vi "MLP_PID_Trajectory tracking_0128.vi"() -> ()   [LabVIEW 2018]
doc: "Demonstrates the use of the Network Streams functions to send LED status to the myRIO target."
uses:
  <vilib>/ErrorRing/Error Ring.xnode
  <vilib>/vision/NI_Vision_Development_Module.lvlib
panel:
  in  "Operation":T1(ring)=enum."Erode"
  out "real_relative_point_y":dbl
  out "real_relative_point_x":dbl
  out "real_relative_start_point_y":dbl
  out "real_relative_start_point_x":dbl
  out "Bounding Box.Y Top 2":i32
  out "Bounding Box.X Left 2":i32
  out "Ki part":dbl
  out "Kd part":dbl
  out "Kp part":dbl
  out "Ki part":dbl
  out "Kd part":dbl
  out "Kp part":dbl
  in  "Ki":dbl=0.02
  in  "Kd":dbl=1e-05
  in  "Kp":dbl=0.003
  in  "Ki":dbl=0.02
  in  "Kd":dbl=1e-05
  in  "Kp":dbl=0.008
  out "添加的数组":dbl[](array[numeric])
  out "desired_relative_point_y":dbl
  out "desired_relative_point_x":dbl
  out "predicted_output_pr":dbl
  out "predicted_output_dr":dbl
  out "error_relative_point_y":dbl
  out "error_relative_point_x":dbl
  out "real_relative_end_point_y":dbl
  out "real_relative_end_point_x":dbl
  out "magnet_input_pr":dbl
  out "magnet_input_dr":dbl
  in  "打开仅尖端轨迹":bool
  out "仅尖端轨迹":T2(plugin-control)
  out "Bounding Box.Y Top":i32
  out "Bounding Box.X Left":i32
  out "curve_min_y":dbl
  out "curve_min_x":dbl
  out "curve_max_y":dbl
  out "curve_max_x":dbl
  out "relative_end_point_y":dbl
  out "relative_end_point_x":dbl
  out "delta_y":dbl
  out "delta_x":dbl
  out "pr":dbl
  out "tan(v)":dbl
  out "delta_velocity":dbl format="%#_10g"
  out "delta_time":dbl
  out "now time":timestamp[](array[timestamp])
  out "prev time":timestamp[](array[timestamp])
  out "delta_distance":dbl
  out "prev_end_point_y":dbl
  out "prev_end_point_x":dbl
  out "now_end_point_y":dbl
  out "now_end_point_x":dbl
  out "prev_end_point_y":dbl[](array[numeric])
  out "prev_end_point_x":dbl[](array[numeric])
  out "dr":dbl
  in  "Ar":sgl=11.0
  out "all parameters":dbl[][](array[numeric])
  out "direction angle":sgl[](array[numeric])
  out "dr":sgl
  out "strength":dbl[](array[numeric])
  out "场强":dbl
  out "end_point_y":T3
  out "end_point_x":dbl[](array[numeric])
  out "start_point_y":dbl[](array[numeric])
  out "start_point_x":dbl[](array[numeric])
  out "T":i32[](array[numeric])
  out "c":dbl[](array[numeric])
  out "b":dbl[](array[numeric])
  out "a\na":dbl[](array[numeric])
  out "c":dbl
  out "b":dbl
  out "a":dbl
  out "Angles (deg)":sgl[](array[numeric]) format="%.2f"
  in  "wr":sgl
  in  "打开轨迹":bool
  out "中心轨迹和尖端轨迹":T2(plugin-control)
  out "end_y":dbl
  out "end_x":dbl
  out "start_y":dbl
  out "start_x":dbl
  out "Image Pixels (U8)":u8[][](array[numeric])
  in  "Poly":dbl
  out "中心轨迹":T2(plugin-control)
  in  "保存按钮":bool
  out "Object Center":cluster{"X":sgl, "Y":sgl}
  out "黑白图":T2(plugin-control)
  in  "Number of Erosion":i32=5
  in  "Settings":T4={"Objects"=1, "Threshold"=128, "Reject Border"=FALSE, "Fill Holes"=FALSE, "Min Object Size"=TRUE, "Min Size"=5500, "Max Object Size"=FALSE, "Max Size"=100, "Show Search Area"=TRUE, "Show Center"=TRUE, "Show Bounding Box"=TRUE} {"Objects" items=["Bright Objects", "Dark Objects"]; "Threshold" min=1 max=999999999 step=1; "Max Size" min=1 max=999999999 step=1; "Min Size" min=1 max=999999999 step=1}
  out "Objects":T5(array[cluster]) {"Aspect Ratio" format="%.2f"; "Orientation" format="%.2f"; "Area" format="%.2f"; "Object Center"."Y" format="%.2f"; "Object Center"."X" format="%.2f"}
  in  "Search Rect (entire image)":T6={"Left"=160, "Top"=740, "Right"=1900, "Bottom"=1620, "Rotation"=0.0} {"Rotation" format="%.2f"; "Left" scale=0.0..1024.0; "Right" scale=0.0..1024.0}
  in  "Range":cluster{"Lower value":sgl, "Upper value":sgl}={"Lower value"=170.0, "Upper value"=255.0} {"Upper value" format="%.2f"; "Lower value" format="%.2f"}
  out "原图":T2(plugin-control)
  in  "停止":bool
  out "T":i32
  out "T":i32
  in  "磁场变换":bool=TRUE
  in  "Pause":bool
  out "Array":dbl[](array[numeric])
  in  "Parameter Settings":T7(tab)=enum."Rotating Field" caption="Field Types"
  in  "Ag":dbl
  in  "dg":dbl
  in  "pg":dbl
  in  "fg":dbl
  in  "AoOF":dbl
  in  "fo":sgl
  in  "do":sgl
  in  "oo":sgl
  in  "po":sgl
  in  "cc":sgl
  in  "pc":sgl
  in  "wc":sgl
  in  "dc":sgl
  in  "Ac":dbl
  in  "Dis phase step":dbl
  in  "Dis phase frequency (Hz)":dbl
  in  "Dis tumbling frequency (Hz)":dbl
  in  "Dis strength(mT)":dbl
  in  "Swa strength (mT)":dbl
  in  "Swa frequency (Hz)":dbl
  in  "Swa pitch angle (deg)":dbl
  in  "Swa direction angle (deg)":dbl
  in  "Swa ratio":dbl=1.0
  in  "Pitch Angle (rotating around Constant, deg)":dbl
  in  "Ratio (A/C)":sgl
  in  "Direction Angle (deg)":sgl
  in  "Pitch Angle (rotating around Origin, deg)":sgl
  in  "Frequency (Hz)":sgl
  in  "Strength (mT)":dbl
  in  "Ar 2":dbl caption="Ar"
  in  "ratio":sgl
  in  "pr  2":sgl
  in  "dr  2":sgl
  in  "wr  2":sgl
  in  "p_x":sgl
  out "Numeric 5":i32
  in  "Stop":bool
  out "error out":errorcluster
  in  "Target IP Address":string="172.22.11.2"
  # "Overview: Magnetic field calculation, and send parameters to myRIO\nInstructions:\n1. Verify the value of Target IP Address. Set Visa resource name.\n2. Ensure RT Main.vi is already running. \n3. Run this VI. Set parameters of magnetic field."
  # "Strength (mT)"
  # "Frequency (Hz)"
  # "Pitch Angle (deg)"
  # "Direction Angle (deg)"
  # "Strength (mT)"
  # "Pitch Angle (deg)"
  # "Direction Angle (deg)"
  # "Frequency (Hz)"
  # "Strength (mT)"
  # "Oscilation Frequency (Hz)"
  # "Oscilation Angle (deg)"
  # "Pitch Angle (deg)"
  # "Direction Angle (deg)"
  # "Strength (mT)"
  # "Frequency (Hz)"
  # "Pitch Angle (deg)"
  # "Direction Angle (deg)"
  # "Conical Angle (deg)"
  # "Strength (mT)"
  # "Tumbling Frequency (Hz)"
  # "Phase Frequency (Hz)"
  # "Phase Step"
  # "Strength (mT)"
  # "Frequency (Hz)"
  # "Pitch Angle (deg)"
  # "Direction Angle (deg)"
  # "Ratio"
  # "Strength (mT)"
  # "Frequency (Hz)"
  # "Ratio (A/C)"
  # "Direction Angle (deg)"
  # "Pitch Angle (rotating around Origin, deg)"
  # "Pitch Angle (rotating around Constant, deg)"
  # "Strength (mT)"
  # "Frequency (Hz)"
  # "Pitch Angle Y (deg)"
  # "Pitch Angle X (deg)"
  # "Direction Angle (deg)"
  # "ratio (l/s)"
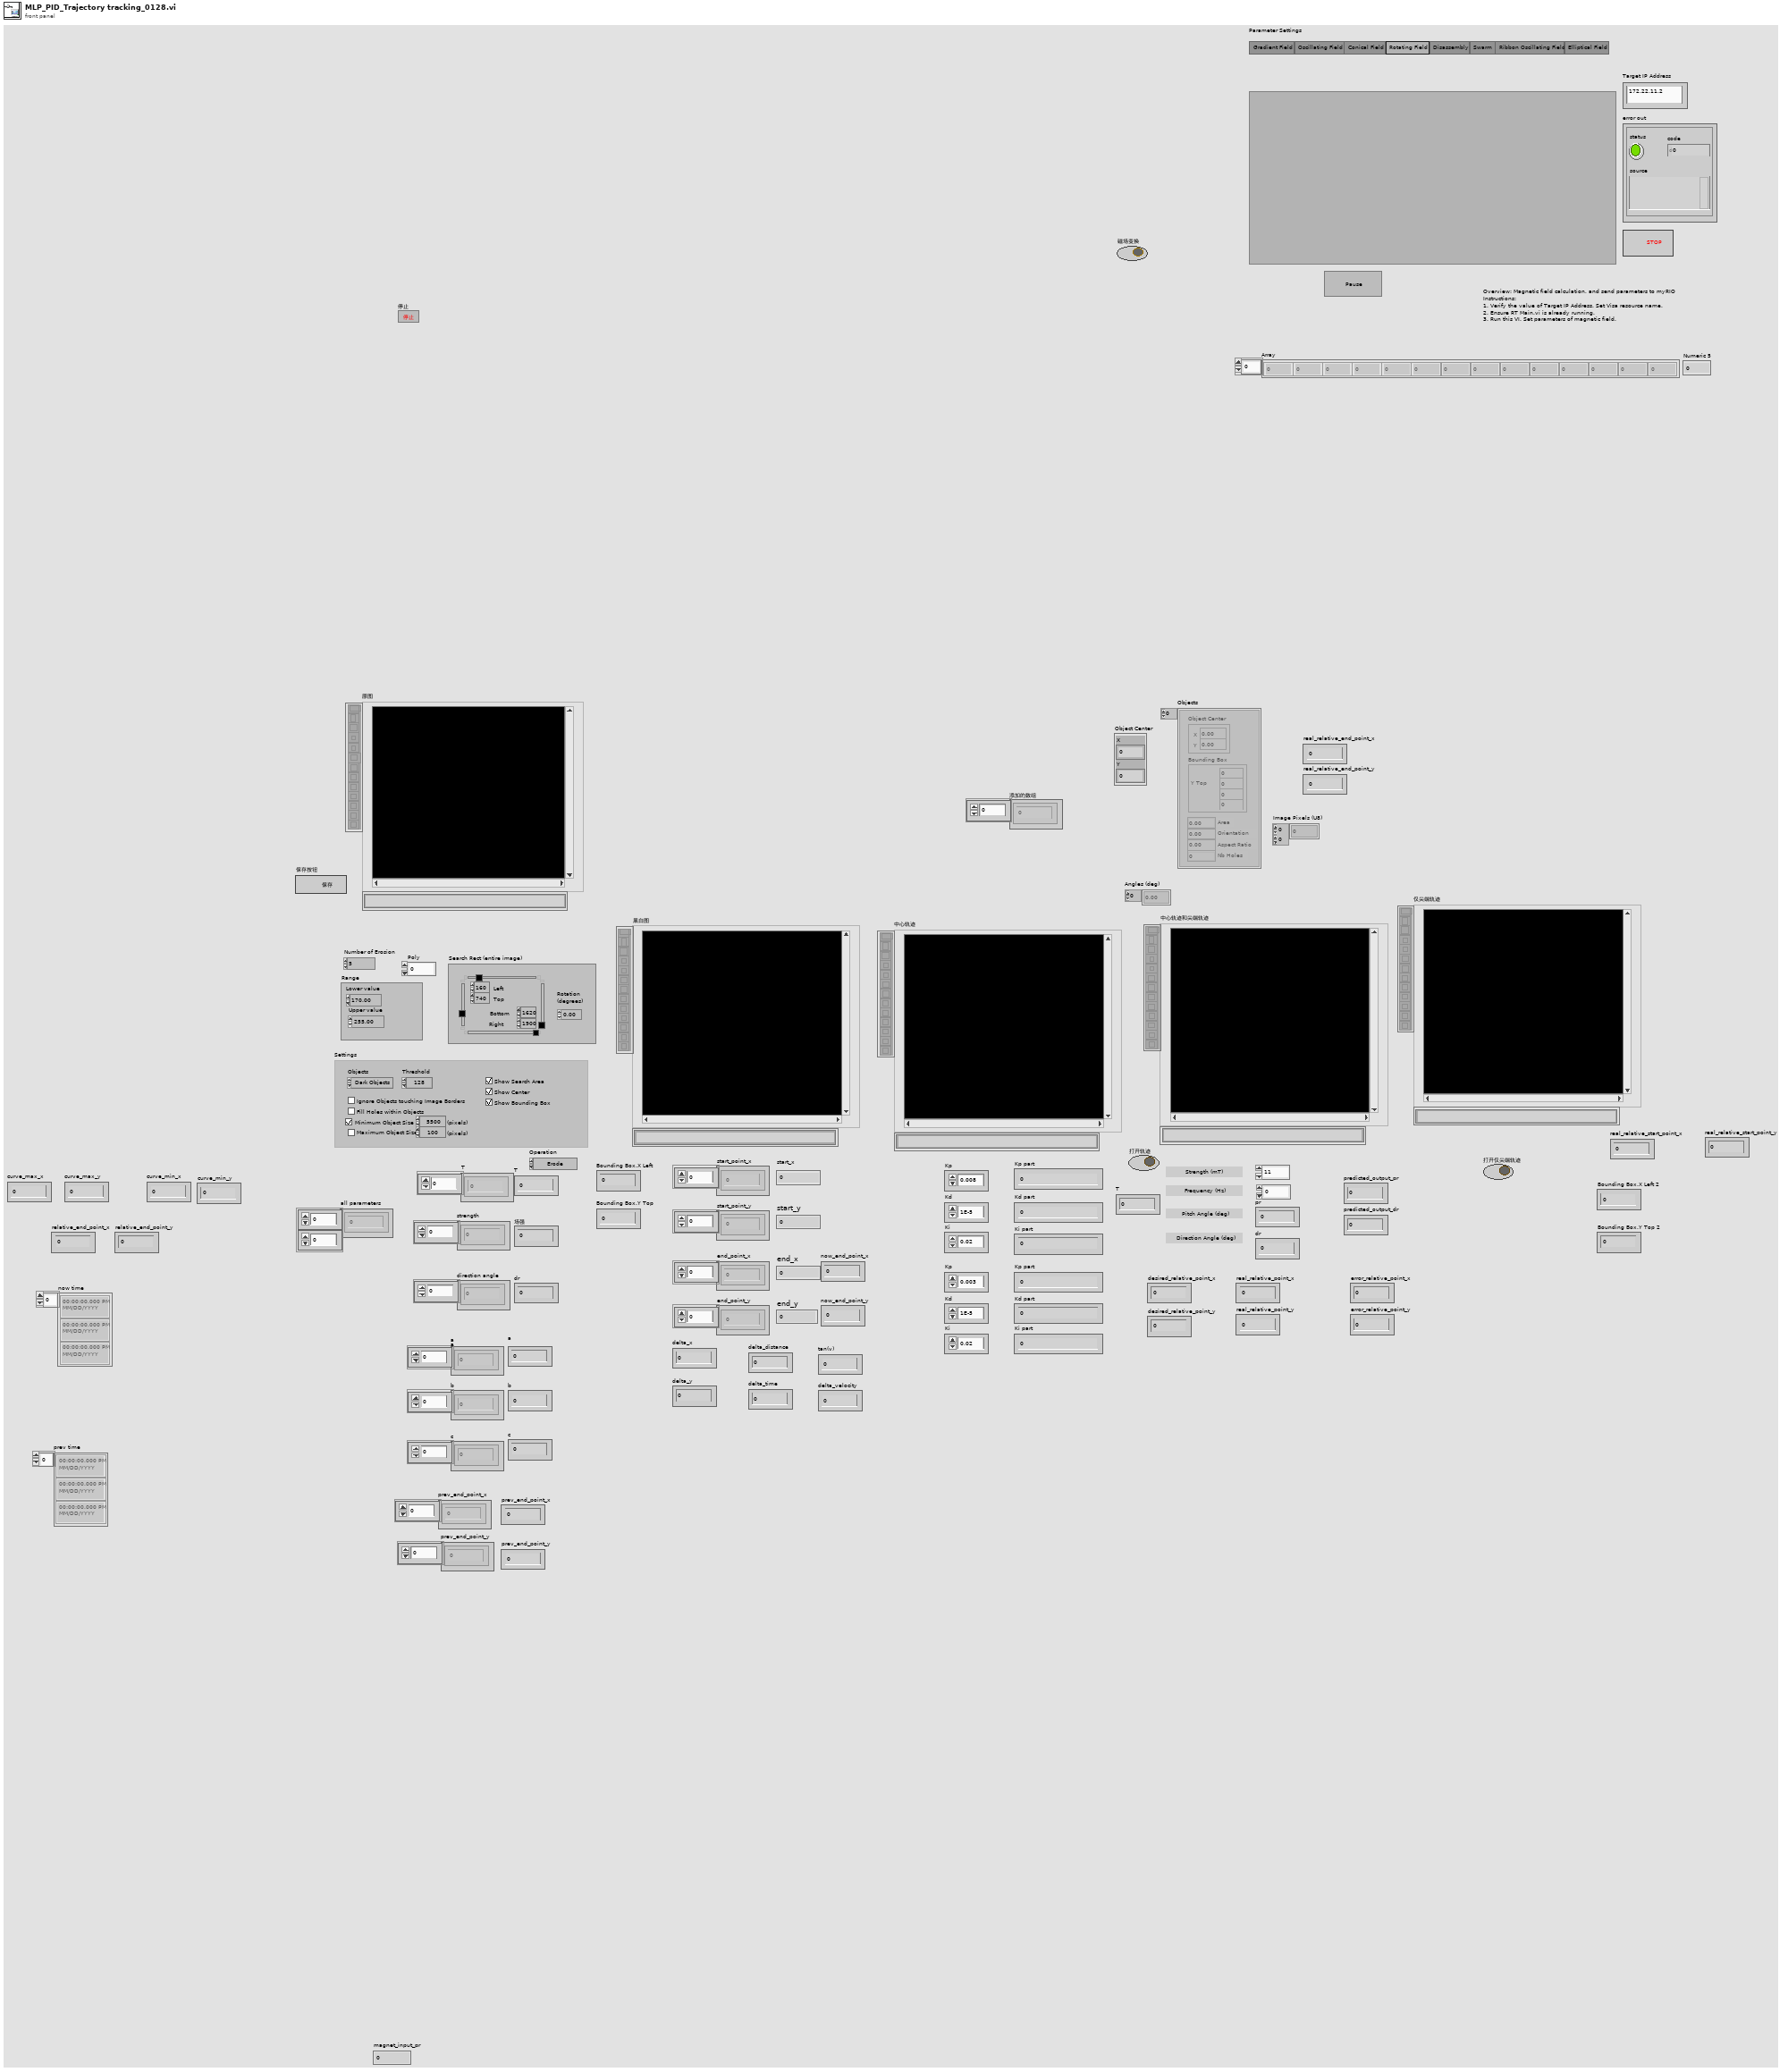
[diagram p1: front panel]
types:
  T1 = enum32{"AutoM", "Close", "Dilate", "Erode", "Gradient", "Gradient in", "Gradient out", "HitMiss", "Open", "PClose", "POpen", "Thick", "Thin"}
  T2 = typedef "IMAQ Image.ctl" = refnum<image>
  T3 = typedef "控件 3.ctl" = dbl[]
  T4 = cluster{"Objects":u16, "Threshold":i32, "Reject Border":bool, "Fill Holes":bool, "Min Object Size":bool, "Min Size":i32, "Max Object Size":bool, "Max Size":i32, "Show Search Area":bool, "Show Center":bool, "Show Bounding Box":bool}
  T5 = cluster{"Object Center":cluster{"X":sgl, "Y":sgl}, "Bounding Box":cluster{"X Left":i32, "Y Top":i32, "X Right":i32, "Y Bottom":i32}, "Area":sgl, "Orientation":sgl, "Aspect Ratio":sgl, "Nb Holes":i32}[]
  T6 = typedef "IMAQ Rectangle" = cluster{"Left":i32, "Top":i32, "Right":i32, "Bottom":i32, "Rotation":dbl}
  T7 = enum32{"Gradient Field ", "Oscillating Field", "Conical Field", "Rotating Field", "Disassembly", "Swarm", "Ribbon Oscillating Field", "Elliptical Field"}
  T8 = typedef "Image Type" = u32
  T9 = cluster{"Object Center":cluster{"X":sgl, "Y":sgl}, "Bounding Box":cluster{"X Left":i32, "Y Top":i32, "X Right":i32, "Y Bottom":i32}, "Area":sgl, "Orientation":sgl, "Aspect Ratio":sgl, "Nb Holes":i32}
  T10 = cluster{"X Left":i32, "Y Top":i32, "X Right":i32, "Y Bottom":i32, "Rotation":dbl}
  T11 = typedef "ROI Descriptor" = cluster{"Global Rectangle":i32[], "Contours":cluster{"ID":enum32{"External", "Internal"}, "Type":u32, "Coordinates":i32[]}[]}
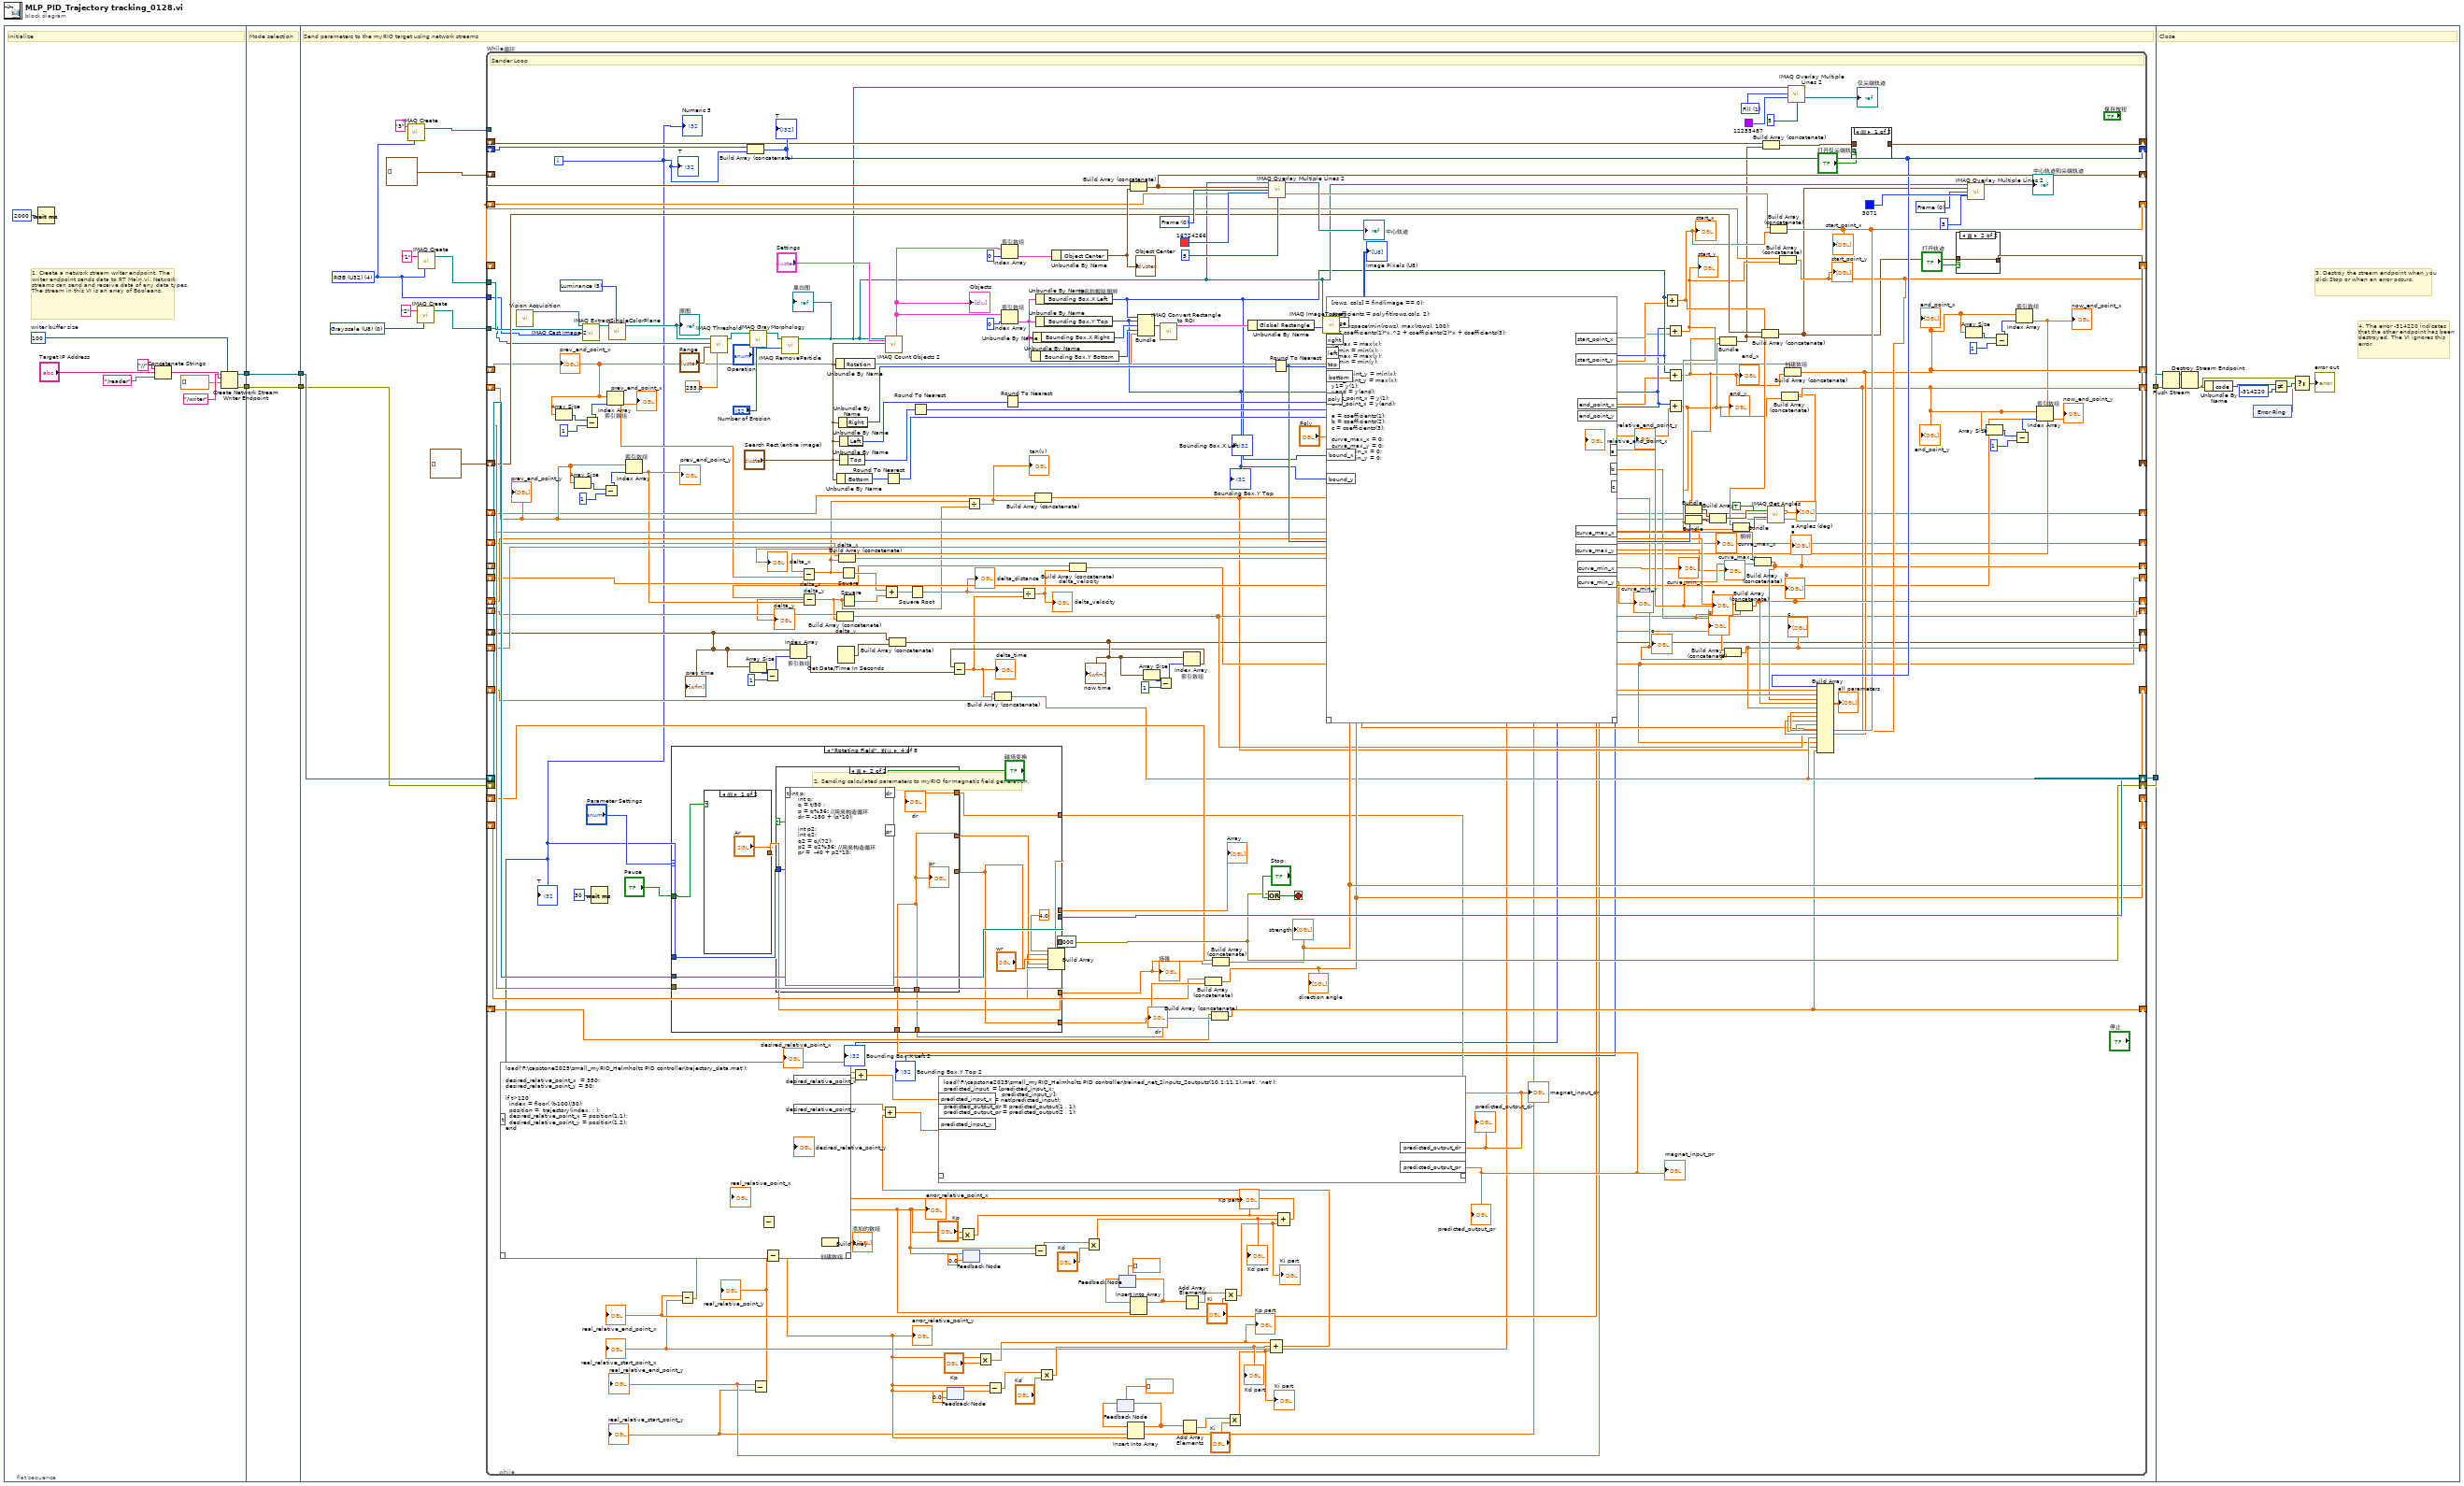
[diagram p0: block diagram]
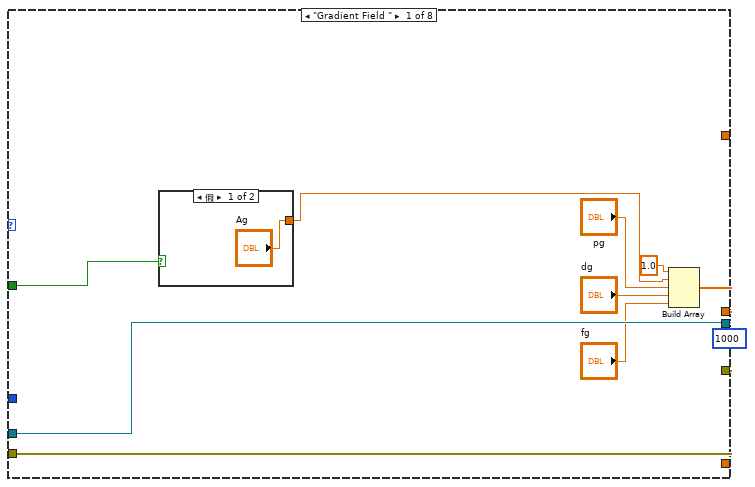
[diagram p4: hidden frame]
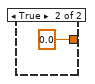
[diagram p5: hidden frame]
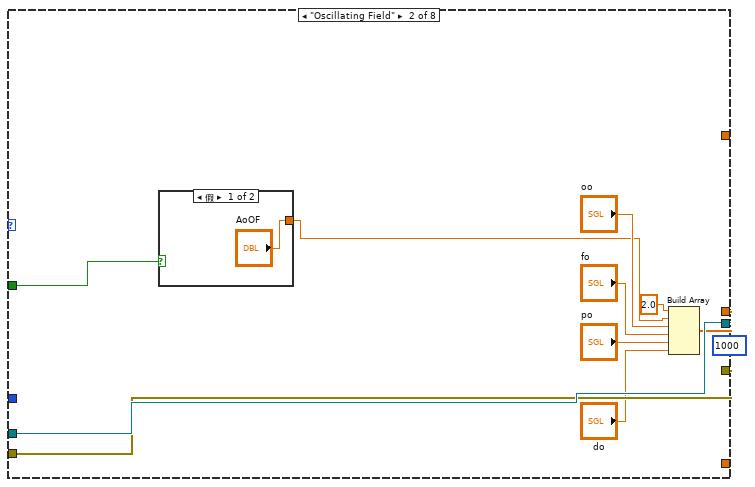
[diagram p6: hidden frame]
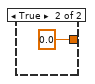
[diagram p7: hidden frame]
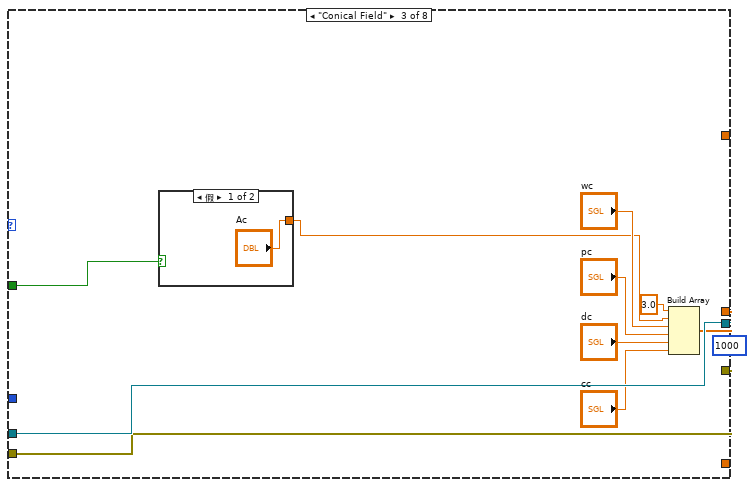
[diagram p8: hidden frame]
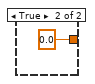
[diagram p9: hidden frame]
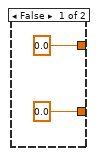
[diagram p10: hidden frame]
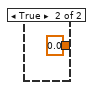
[diagram p11: hidden frame]
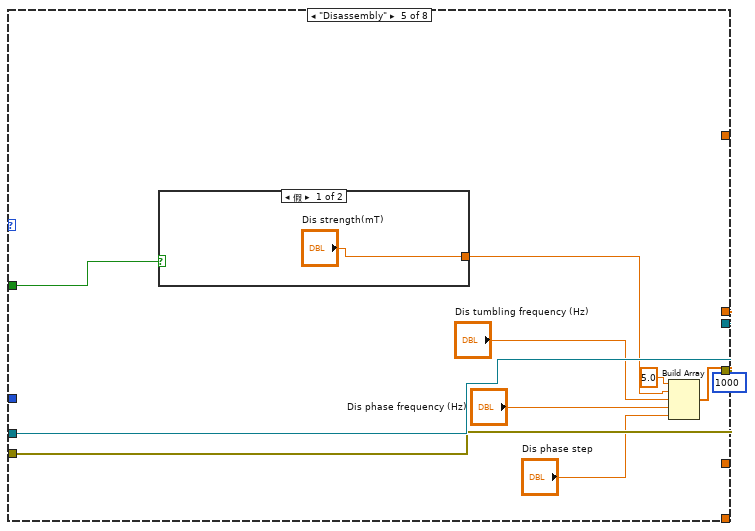
[diagram p12: hidden frame]
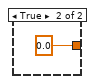
[diagram p13: hidden frame]
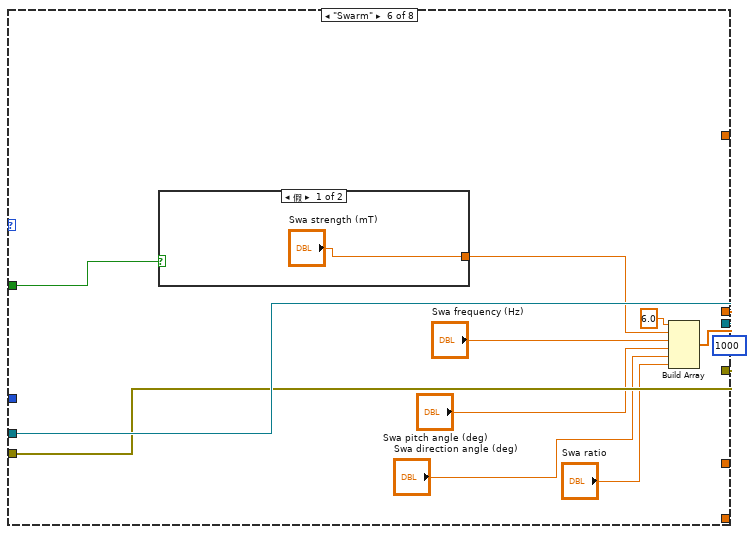
[diagram p14: hidden frame]
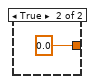
[diagram p15: hidden frame]
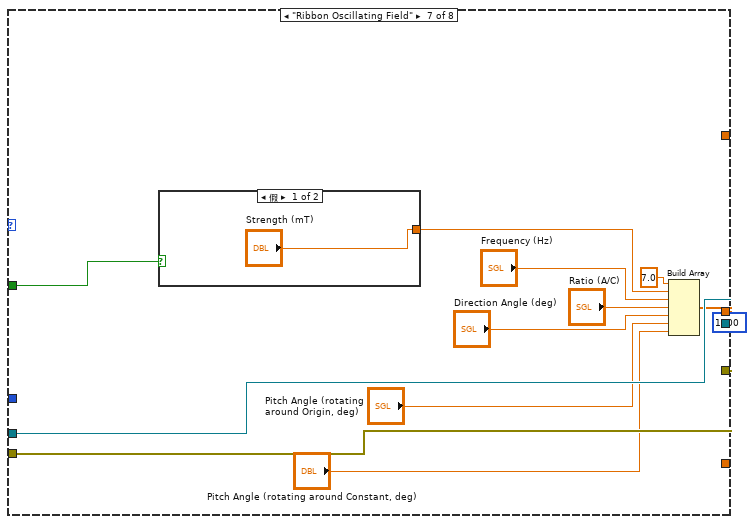
[diagram p16: hidden frame]
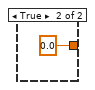
[diagram p17: hidden frame]
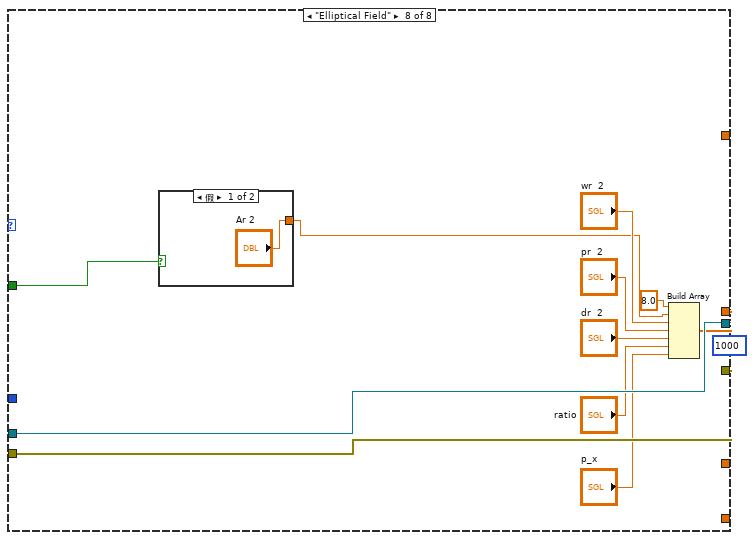
[diagram p18: hidden frame]
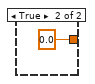
[diagram p19: hidden frame]
diagram:
  n1 = flat-sequence {
    tunnel: [w11] -> w2
    tunnel: [w10] -> w1
    tunnel: [w18] -> w4
    tunnel: [w17] -> w3
    tunnel: w1 -> [w17]
    tunnel: w2 -> [w18]
    tunnel: [w30] -> w6
    tunnel: w4 -> [w32]
    tunnel: [w29] -> w5
    tunnel: w3 -> [w31]
    tunnel: w6 -> [w379]
    tunnel: w5 -> [w376]
    frame #0 {
      w9 = 100  # writer buffer size
      # "1. Create a network stream writer endpoint. The writer endpoint sends data to RT Main.vi. Network streams can send and receive data of any data types. The stream in this VI is an array of Booleans."
      # "Initialize"
      n2 = Wait (ms)(milliseconds to wait=2000) -> ()  [unwired: 1 out]
      n3 = Concatenate Strings("//", "Target IP Address", "/reader") -> (w16:string)
      n4 = Create Network Stream Writer Endpoint(7:w9, 9:dbl[] [], 10:w16, 11:"/writer" ("reader name")) -> (0:w10:errorcluster, 3:w11:refnum<k21>)  [unwired: 3 in]
    }
    frame #1 {
      # "Mode selection"
    }
    frame #2 {
      w26 = T8 0 items=["Grayscale (U8)", "Grayscale (I16)", "Grayscale (SGL)", "Complex (CSG)", "RGB (U32)", "HSL (U32)", "RGB (U64)", "Grayscale (U16)"] ("Image Type")
      w19 = T8 4 items=["Grayscale (U8)", "Grayscale (I16)", "Grayscale (SGL)", "Complex (CSG)", "RGB (U32)", "HSL (U32)", "RGB (U64)", "Grayscale (U16)"] ("Image Type")
      # "Send parameters to the myRIO target using network streams"
      n5 = call "IMAQ Create"("Image Name"="3", "Image Type"=w19) -> ("New Image"=w22:T2)  [unwired: 3 in, 1 out]
      n6 = call "IMAQ Create"("Image Name"="2", "Image Type"=w26) -> ("New Image"=w24:T2)  [unwired: 3 in, 1 out]
      n7 = call "IMAQ Create"("Image Name"="1", "Image Type"=w19) -> ("New Image"=w25:T2)  [unwired: 3 in, 1 out]
      n8 = while "While循环" {
        shift-right: [w234] -> w29
        shift-left: w31 -> [w236]
        shift-right: [w235] -> w30
        shift-left: w32 -> [w237]
        tunnel: w25 -> [w188]
        tunnel: w24 -> [w187]
        tunnel: w22 -> [_]
        shift-right: [w184] -> _
        shift-left: cluster{"X":dbl, "Y":dbl}[] [] -> [w189]
        shift-right: [w190] -> _
        shift-left: cluster{"X":dbl, "Y":dbl}[] [] -> [w191]
        tunnel: w19 -> [w186]
        shift-right: [w156] -> _
        shift-left: _ -> [w176]
        shift-right: [w151] -> _
        shift-left: _ -> [w174]
        shift-right: [w155] -> _
        shift-left: _ -> [w171]
        shift-right: [w159] -> _
        shift-left: _ -> [w170]
        shift-right: [w154] -> _
        shift-left: _ -> [w168]
        shift-right: [w153] -> _
        shift-left: _ -> [w166]
        shift-right: [w147] -> _
        shift-left: _ -> [w139]
        shift-right: [w143] -> _
        shift-left: _ -> [w135]
        shift-right: [w158] -> _
        shift-left: _ -> [w162]
        shift-right: [w157] -> _
        shift-left: _ -> [w160]
        shift-right: [w124] -> _
        shift-left: _ -> [w126]
        shift-right: [w123] -> _
        shift-left: _ -> [w125]
        shift-right: [w113] -> _
        shift-left: _ -> [w118]
        shift-right: [w110] -> _
        shift-left: _ -> [w111]
        shift-right: [w106] -> _
        shift-left: _ -> [w107]
        shift-right: [w101] -> _
        shift-left: _ -> [w102]
        shift-right: [w93] -> _
        shift-left: _ -> [w94]
        shift-right: [w87] -> _
        shift-left: _ -> [w88]
        i -> [w81]
        stop <- w230 stop-if-true
        w89 = u32 1 items=["Frame", "Fill"] ("Drawing Mode (Frame)")
        w96 = u32 0 items=["Frame", "Fill"] ("Drawing Mode (Frame)")
        w217 = u32 0 items=["Frame", "Fill"] ("Drawing Mode (Frame)")
        w227 = 5 items=["Red", "Green", "Blue", "Hue", "Saturation", "Luminance", "Value", "Intensity"] ("Color Plane")
        # "2. Sending calculated parameters to myRIO for magnetic field generation."
        # "Sender Loop"
        n9 = script code="load('F:\\capstone2025\\small_myRIO_Helmholtz PID controller\\trajectory_data.mat');\n\ndesired_relative_point_x  = 350;\ndesired_relative_point_y = 50;\n\nif t>120\n  index = floor( (t-100)/30);\n  position =  trajectory(index, : );\n  desired_relative_point_x = position(1,1);\n  desired_relative_point_y = position(1,2);\nend"("t"=w81) -> ("desired_relative_point_x"=w37:dbl, "desired_relative_point_y"=w36:dbl)  [unwired: 1 in, 1 out]
        "desired_relative_point_x" <- w37
        "desired_relative_point_y" <- w36
        n10 = call "Vision Acquisition"() -> ("Image Out"=w215:T2)  [unwired: 23 in, 4 out]
        n11 = Array Size(array=w139) -> (size(s)=w141:i32)
        n12 = Array Size(array=w135) -> (size(s)=w137:i32)
        n13 = call "IMAQ Cast Image 2"("Image Src"=w215, "Image Dst"=w188, "Image Type"=w186) -> ("Image Dst Out"=w228:T2)  [unwired: 11 in, 1 out]
        n14 = Subtract(x=w141, y=1) -> (x-y=w140:i32)
        n15 = Wait (ms)(milliseconds to wait=u32 30 ("等待时间（毫秒）")) -> ()  [unwired: 1 out]
        n16 = Subtract(x=w137, y=1) -> (x-y=w136:i32)
        n17 = Index Array "索引数组"(array=w139, index=w140) -> (element=w133:dbl)
        "prev_end_point_x" <- w133
        n18 = call "IMAQ ExtractSingleColorPlane"("Color Plane"=w227, "Image Src"=w228) -> ("Image Dst Out"=w226:T2)  [unwired: 8 in, 1 out]
        "原图" <- w226
        n19 = Index Array "索引数组"(array=w135, index=w136) -> (element=w132:dbl)
        "prev_end_point_y" <- w132
        n20 = call "IMAQ Threshold"("Replace Value"=sgl 255.0, "Range"="Range", "Image Dst"=w187, "Image Src"=w226) -> ("Image Dst Out"=w35:T2)  [unwired: 6 in, 1 out]
        n21 = Build Array (concatenate)(w170, w81) -> (w159:i32[])
        "T" <- w159
        n22 = call "IMAQ GrayMorphology"("Operation"="Operation", "Image Src"=w35) -> ("Image Dst Out"=w34:T2)  [unwired: 8 in, 1 out]
        n23 = Array Size(array=w118) -> (size(s)=w121:i32)
        n24 = Subtract(x=w121, y=1) -> (x-y=w120:i32)
        n25 = call "IMAQ RemoveParticle"("Number of Erosion"="Number of Erosion", "Image Src"=w34) -> ("Image Dst Out"=w85:T2)  [unwired: 8 in, 1 out]
        "黑白图" <- w85
        n26 = Index Array "索引数组"(array=w118, index=w120) -> (element=w117:timestamp)
        n27 = Unbundle By Name("Search Rect (entire image)") -> ("Rotation"=w212:dbl)
        n28 = Unbundle By Name("Search Rect (entire image)") -> ("Bottom"=w196:i32)
        n29 = Get Date/Time In Seconds() -> (seconds since 1Jan1904=w122:timestamp)
        n30 = Unbundle By Name("Search Rect (entire image)") -> ("Right"=w200:i32)
        n31 = Unbundle By Name("Search Rect (entire image)") -> ("Left"=w199:i32)
        n32 = Unbundle By Name("Search Rect (entire image)") -> ("Top"=w198:i32)
        n33 = Round To Nearest(number=w196) -> (nearest integer value=w195:i32)
        n34 = call "IMAQ Count Objects 2"("Settings"="Settings", "Search Rect (entire image)"="Search Rect (entire image)", "Image"=w85) -> ("Objects"=w214:T5)  [unwired: 4 in, 4 out]
        "Objects" <- w214
        n35 = Build Array (concatenate)(w118, w122) -> (w113:timestamp[])
        "now time" <- w113
        n36 = Round To Nearest(number=w198) -> (nearest integer value=w197:i32)
        n37 = feedback #1(0.0) -> (w63:dbl)
        n38 = feedback #2(0.0) -> (w77:dbl)
        n39 = Index Array "索引数组"(array=w214, index=0 ("索引")) -> (element=w220:T9)
        n40 = Index Array "索引数组"(array=w214, index=0 ("索引")) -> (element=w210:T9)
        n41 = Round To Nearest(number=w199) -> (nearest integer value=w193:i32)
        n42 = Unbundle By Name(w210) -> ("Bounding Box.Y Bottom"=w204:i32)
        n43 = Unbundle By Name(w210) -> ("Bounding Box.X Right"=w205:i32)
        n44 = Unbundle By Name "按名称解除捆绑"(w210) -> ("Bounding Box.X Left"=w45:i32)
        "Bounding Box.X Left" <- w45
        "Bounding Box.X Left 2" <- w45
        n45 = Unbundle By Name(w210) -> ("Bounding Box.Y Top"=w44:i32)
        "Bounding Box.Y Top" <- w44
        "Bounding Box.Y Top 2" <- w44
        n46 = Unbundle By Name(w220) -> ("Object Center"=w219:cluster{"X":sgl, "Y":sgl})
        "Object Center" <- w219
        n47 = feedback #3(dbl[] []) -> (w58:dbl[])
        n48 = feedback #4(dbl[] []) -> (w72:dbl[])
        n49 = Build Array (concatenate)(w191, w219) -> (w190:cluster{"X":dbl, "Y":dbl}[])
        n50 = Bundle("X Left"=w45, "Y Top"=w44, "X Right"=w205, "Y Bottom"=w204, "Rotation"=w212) -> (w211:T10)  [unwired: 1 in]
        n51 = Array Size(array=w113) -> (size(s)=w116:i32)
        n52 = Subtract(x=w116, y=1) -> (x-y=w115:i32)
        n53 = call "IMAQ Convert Rectangle to ROI"("Rectangle"=w211) -> ("ROI Descriptor"=w209:T11)  [unwired: 8 in, 1 out]
        n54 = Index Array "索引数组"(array=w113, index=w115) -> (element=w112:timestamp)
        n55 = Subtract(x=w112, y=w117) -> (x-y=w109:dbl)
        "delta_time" <- w109
        n56 = Build Array (concatenate)(w111, w109) -> (w110:dbl[])
        n57 = Unbundle By Name(w209) -> ("Global Rectangle"=w194:i32[])
        n58 = call "IMAQ Overlay Multiple Lines 2"("Image"=w85, "Line End Points"=w190, "Drawing Mode (Frame)"=w217, "Color"=u32 16724266, "Width"=u32 5) -> ("Image Out"=→"中心轨迹":T2)  [unwired: 9 in, 1 out]
        n59 = Round To Nearest(number=w200) -> (nearest integer value=w177:i32)
        n60 = call "IMAQ ImageToArray"("Optional Rectangle"=w194, "Image"=w85) -> ("Image Pixels (U8)"=w206:u8[][])  [unwired: 2 in, 4 out]
        "Image Pixels (U8)" <- w206
        n61 = script code="[rows, cols] = find(image == 0); \n\ncoefficients = polyfit(rows,cols, 2);\n\nx = linspace(min(rows), max(rows), 100); \ny = coefficients(1)*x.^2 + coefficients(2)*x + coefficients(3);\n\nx_max = max(x);\nx_min = min(x);\ny_max = max(y);\ny_min = min(y);\n\nstart_point_y = min(x);\nend_point_y = max(x);\ny1= y(1);\nyend = y(end);\nstart_point_x = y(1);\nend_point_x = y(end);\n\na = coefficients(1);\nb = coefficients(2);\nc = coefficients(3);\n\ncurve_max_x = 0;\ncurve_max_y = 0;\ncurve_min_x = 0;\ncurve_min_y = 0;"("image"=w206, "poly"="Poly", "right"=w177, "left"=w193, "top"=w197, "bottom"=w195, "bound_x"=w45, "bound_y"=w44) -> ("start_point_x"=w42:dbl, "start_point_y"=w39:dbl, "end_point_x"=w43:dbl, "end_point_y"=w40:dbl, "a"=w175:dbl, "b"=w173:dbl, "c"=w172:dbl, "curve_max_x"=→"curve_max_x":dbl, "curve_max_y"=→"curve_max_y":dbl, "curve_min_x"=→"curve_min_x":dbl, "curve_min_y"=→"curve_min_y":dbl)  [unwired: 1 in, 1 out]
        "a" <- w175
        "b" <- w173
        "c" <- w172
        "relative_end_point_x" <- w43
        "relative_end_point_y" <- w40
        "real_relative_end_point_x" <- w43
        "real_relative_end_point_y" <- w40
        "real_relative_start_point_x" <- w42
        "real_relative_start_point_y" <- w39
        n62 = Subtract(x=w43, y=w42) -> (x-y=w41:dbl)
        "real_relative_point_x" <- w41
        n63 = Subtract(x=w40, y=w39) -> (x-y=w38:dbl)
        "real_relative_point_y" <- w38
        n64 = Subtract(x=w37, y=w41) -> (x-y=w71:dbl)
        "error_relative_point_x" <- w71
        n65 = Subtract(x=w36, y=w38) -> (x-y=w56:dbl)
        "error_relative_point_y" <- w56
        n66 = Build Array "创建数组"(w71, w56) -> (→"添加的数组":dbl[])
        n67 = feedback-in #1(w56) -> ()
        n68 = Multiply(x=w71, y="Kp") -> (x*y=w78:dbl)
        "Kp part" <- w78
        n69 = feedback-in #2(w71) -> ()
        n70 = Multiply(x=w56, y="Kp") -> (x*y=w64:dbl)
        "Kp part" <- w64
        n71 = Subtract(x=w56, y=w63) -> (x-y=w61:dbl)
        n72 = Subtract(x=w71, y=w77) -> (x-y=w75:dbl)
        n73 = Multiply(x=w61, y="Kd") -> (x*y=w59:dbl)
        "Kd part" <- w59
        n74 = Multiply(x=w75, y="Kd") -> (x*y=w73:dbl)
        "Kd part" <- w73
        n75 = Insert Into Array(array=w58, new element=w56) -> (w57:dbl[])  [unwired: 1 in]
        n76 = feedback-in #3(w57) -> ()
        n77 = Insert Into Array(array=w72, new element=w71) -> (w70:dbl[])  [unwired: 1 in]
        n78 = feedback-in #4(w70) -> ()
        n79 = Add Array Elements(numeric array=w57) -> (sum=w54:dbl)
        n80 = Add Array Elements(numeric array=w70) -> (sum=w68:dbl)
        n81 = Multiply(x=w68, y="Ki") -> (x*y=w66:dbl)
        "Ki part" <- w66
        n82 = Multiply(x=w54, y="Ki") -> (x*y=w52:dbl)
        "Ki part" <- w52
        n83 = Compound Arithmetic op=ADD(w64, w59, w52) -> (w47:dbl)
        n84 = Add(x=w36, y=w47) -> (x+y=w48:dbl)
        n85 = Compound Arithmetic op=ADD(w78, w73, w66) -> (w49:dbl)
        n86 = Add(x=w37, y=w49) -> (x+y=w50:dbl)
        n87 = script code="load('F:\\capstone2025\\small_myRIO_Helmholtz PID controller\\trained_net_2inputs_2outputs(10,1;11,1).mat', 'net');\npredicted_input  = [predicted_input_x; \n                               predicted_input_y];\npredicted_output = net(predicted_input);\npredicted_output_dr = predicted_output(1 , 1);\npredicted_output_pr = predicted_output(2 , 1);"("predicted_input_y"=w48, "predicted_input_x"=w50) -> ("predicted_output_dr"=w46:dbl, "predicted_output_pr"=w51:dbl)  [unwired: 1 in, 1 out]
        "magnet_input_dr" <- w46
        "magnet_input_pr" <- w51
        "predicted_output_dr" <- w46
        "predicted_output_pr" <- w51
        n88 = case shown="\"Rotating Field\", 默认" "Parameter Settings" {
          tunnel: w237 -> [w251 w266 w281 w300 w319 w333 w351 w366]
          tunnel: w236 -> [w248 w265 w280 w299 w317 w332 w349 w365]
          tunnel: [w250 w264 w278 w298 w318 w331 w350 w364] -> w235
          tunnel: [w249 w263 w279 w297 w316 w330 w348 w363] -> w234
          tunnel: [w244 w257 w272 w293 w310 w325 w346 w358] -> w233
          tunnel: "Pause" -> [w242 w255 w270 w292 w309 w324 w341 w356]
          tunnel: [_ _ _ w289 _ _ _ _] -> w163
          tunnel: [_ _ _ w290 _ _ _ _] -> w161
          tunnel: w81 -> [_ _ _ w288 _ _ _ _]
          tunnel: [_ _ _ w287 _ _ _ _] -> w95
          tunnel: w46 -> [_ _ _ w286 _ _ _ _]
          tunnel: w51 -> [_ _ _ w285 _ _ _ _]
          frame "Gradient Field " {
            n89 = case shown="假" w242 {
              tunnel: ["Ag" 0.0] -> w243
              frame False {
              }
              frame True {
              }
            }
            n90 = Build Array(1.0, w243, "pg", "dg", "fg") -> (w244:dbl[])
            n91 = shared-variable-write(w251, w248, w244, 1000 ("timeout ms (-1)")) -> (w250:refnum<k21>, w249:errorcluster)  [unwired: 1 out]
          }
          frame "Oscillating Field" {
            n92 = case shown="假" w255 {
              tunnel: ["AoOF" 0.0] -> w256
              frame False {
              }
              frame True {
              }
            }
            n93 = Build Array(2.0, w256, "oo", "fo", "po", "do") -> (w257:dbl[])
            n94 = shared-variable-write(w266, w265, w257, 1000 ("timeout ms (-1)")) -> (w264:refnum<k21>, w263:errorcluster)  [unwired: 1 out]
          }
          frame "Conical Field" {
            # "FG"
            n95 = case shown="假" w270 {
              tunnel: ["Ac" 0.0] -> w271
              frame False {
              }
              frame True {
              }
            }
            n96 = Build Array(3.0, w271, "wc", "pc", "dc", "cc") -> (w272:dbl[])
            n97 = shared-variable-write(w281, w280, w272, 1000 ("timeout ms (-1)")) -> (w278:refnum<k21>, w279:errorcluster)  [unwired: 1 out]
          }
          frame "Rotating Field", Default {
            n98 = case shown="假" w292 {
              tunnel: ["Ar" 0.0] -> w289
              frame False {
              }
              frame True {
              }
            }
            n99 = case shown="真" "磁场变换" {
              tunnel: [sgl 0.0 ("pr") w304] -> w295
              tunnel: [sgl 0.0 ("dr") w305] -> w290
              tunnel: w288 -> [_ w306]
              tunnel: [_ w304] -> w287
              tunnel: w286 -> [_ w305]
              tunnel: w285 -> [_ w304]
              frame False {
              }
              frame True {
                n100 = formula code="int p;\n    int q;\n    q = t/50 ;  \n    p = q%36; //用来构造循环\n    dr = -180 + (p*10);\n\n    int p2;\n    int q2;\n    q2 = q/(72);\n    p2 = q2%36; //用来构造循环\n    pr =  -40 + p2*10;"("t"=w306) -> ()  [unwired: 2 out]
                "dr" <- w305
                "pr" <- w304
              }
            }
            n101 = Build Array(4.0, w289, "wr", w295, w290) -> (w293:dbl[])
            n102 = shared-variable-write "向流中写入单个元素"(w300, w299, w293, 1000 ("timeout ms (-1)")) -> (w298:refnum<k21>, w297:errorcluster)  [unwired: 1 out]
          }
          frame "Disassembly" {
            n103 = case shown="假" w309 {
              tunnel: ["Dis strength(mT)" 0.0] -> w314
              frame False {
              }
              frame True {
              }
            }
            n104 = Build Array(5.0, w314, "Dis tumbling frequency (Hz)", "Dis phase frequency (Hz)", "Dis phase step") -> (w310:dbl[])
            n105 = shared-variable-write(w319, w317, w310, 1000 ("timeout ms (-1)")) -> (w318:refnum<k21>, w316:errorcluster)  [unwired: 1 out]
          }
          frame "Swarm" {
            n106 = case shown="假" w324 {
              tunnel: ["Swa strength (mT)" 0.0] -> w323
              frame False {
              }
              frame True {
              }
            }
            n107 = Build Array(6.0, w323, "Swa frequency (Hz)", "Swa pitch angle (deg)", "Swa direction angle (deg)", "Swa ratio") -> (w325:dbl[])
            n108 = shared-variable-write(w333, w332, w325, 1000 ("timeout ms (-1)")) -> (w331:refnum<k21>, w330:errorcluster)  [unwired: 1 out]
          }
          frame "Ribbon Oscillating Field" {
            n109 = case shown="假" w341 {
              tunnel: ["Strength (mT)" 0.0] -> w340
              frame False {
              }
              frame True {
              }
            }
            n110 = Build Array(7.0, w340, "Frequency (Hz)", "Ratio (A/C)", "Direction Angle (deg)", "Pitch Angle (rotating around Origin, deg)", "Pitch Angle (rotating around Constant, deg)") -> (w346:dbl[])
            n111 = shared-variable-write(w351, w349, w346, 1000 ("timeout ms (-1)")) -> (w350:refnum<k21>, w348:errorcluster)  [unwired: 1 out]
          }
          frame "Elliptical Field" {
            n112 = case shown="假" w356 {
              tunnel: ["Ar 2" 0.0] -> w357
              frame False {
              }
              frame True {
              }
            }
            n113 = Build Array(8.0, w357, "wr  2", "pr  2", "dr  2", "ratio", "p_x") -> (w358:dbl[])
            n114 = shared-variable-write(w366, w365, w358, 1000 ("timeout ms (-1)")) -> (w364:refnum<k21>, w363:errorcluster)  [unwired: 1 out]
          }
        }
        "Array" <- w233
        "场强" <- w163
        "dr" <- w161
        n115 = Build Array (concatenate)(w160, w161) -> (w157:dbl[])
        "direction angle" <- w157
        n116 = Build Array (concatenate)(w94, w95) -> (w93:dbl[])
        n117 = Build Array (concatenate)(w162, w163) -> (w158:dbl[])
        "strength" <- w158
        n118 = Or(x=w234, y="Stop") -> (x .or. y?=w230:bool)
        n119 = Add(x=w45, y=w42) -> (x+y=w169:dbl)
        "start_x" <- w169
        n120 = Add(x=w44, y=w39) -> (x+y=w167:dbl)
        "start_y" <- w167
        n121 = Add(x=w45, y=w43) -> (x+y=w165:dbl)
        "end_x" <- w165
        n122 = Add(x=w44, y=w40) -> (x+y=w164:dbl)
        "end_y" <- w164
        n123 = Bundle(w165, w164) -> (w181:cluster{dbl, dbl})  [unwired: 1 in]
        n124 = Bundle(w177, w167) -> (w180:cluster{i32, dbl})  [unwired: 1 in]
        n125 = Build Array(w181, w180) -> (w179:cluster{dbl, dbl}[])
        n126 = Bundle(w165, w164) -> (w83:cluster{dbl, dbl})  [unwired: 1 in]
        n127 = Build Array (concatenate)(w171, w172) -> (w155:dbl[])
        "c" <- w155
        n128 = Bundle "捆绑"(w169, w167) -> (w182:cluster{dbl, dbl})  [unwired: 1 in]
        n129 = Build Array (concatenate)(w174, w173) -> (w151:dbl[])
        "b" <- w151
        n130 = Build Array (concatenate)(w176, w175) -> (w156:dbl[])
        "a\na" <- w156
        n131 = Build Array (concatenate)(w189, w83) -> (w84:cluster{"X":dbl, "Y":dbl}[])
        n132 = Build Array (concatenate)(w88, w83) -> (w82:cluster{dbl, dbl}[])
        n133 = call "IMAQ Get Angles"("Vertex"=w182, "Points"=w179, "Use Vertex (No)"=TRUE) -> ("Angles (deg)"=→"Angles (deg)":sgl[])  [unwired: 2 in, 2 out]
        n134 = Build Array (concatenate)(w168, w169) -> (w154:dbl[])
        "start_point_x" <- w154
        n135 = Build Array (concatenate)(w166, w167) -> (w153:dbl[])
        "start_point_y" <- w153
        n136 = Build Array (concatenate)(w135, w164) -> (w143:dbl[])
        "end_point_y" <- w143
        n137 = Build Array (concatenate) "创建数组"(w139, w165) -> (w147:dbl[])
        "end_point_x" <- w147
        n138 = call "IMAQ Overlay Multiple Lines 2"("Image"=w85, "Drawing Mode (Frame)"=w89, "Color"=u32 12255487, "Width"=u32 5) -> ("Image Out"=→"仅尖端轨迹":T2)  [unwired: 10 in, 1 out]
        n139 = case shown="假" "打开仅尖端轨迹" {
          tunnel: [_ w239] -> w87
          tunnel: w82 -> [_ w239]
          frame False {
          }
          frame True {
          }
        }
        n140 = case shown="真" "打开轨迹" {
          tunnel: [_ w240] -> w184
          tunnel: w84 -> [_ w240]
          frame False {
          }
          frame True {
          }
        }
        n141 = Array Size(array=w147) -> (size(s)=w149:i32)
        n142 = call "IMAQ Overlay Multiple Lines 2"("Image"=w85, "Line End Points"=w84, "Drawing Mode (Frame)"=w96, "Color"=u32 3071, "Width"=u32 5) -> ("Image Out"=→"中心轨迹和尖端轨迹":T2)  [unwired: 9 in, 1 out]
        n143 = Array Size(array=w143) -> (size(s)=w145:i32)
        n144 = Subtract(x=w149, y=1) -> (x-y=w148:i32)
        n145 = Subtract(x=w145, y=1) -> (x-y=w144:i32)
        n146 = Index Array "索引数组"(array=w147, index=w148) -> (element=w134:dbl)
        "now_end_point_x" <- w134
        n147 = Subtract "delta_x"(x=w134, y=w133) -> (x-y=w105:dbl)
        "delta_x" <- w105
        n148 = Build Array (concatenate) "delta_x"(w126, w105) -> (w124:dbl[])
        n149 = Square(x=w105) -> (x^2=w130:dbl)
        n150 = Index Array "索引数组"(array=w143, index=w144) -> (element=w131:dbl)
        "now_end_point_y" <- w131
        n151 = Subtract "delta_y"(x=w131, y=w132) -> (x-y=w104:dbl)
        "delta_y" <- w104
        n152 = Build Array (concatenate) "delta_y"(w125, w104) -> (w123:dbl[])
        n153 = Square(x=w104) -> (x^2=w129:dbl)
        n154 = Add(x=w130, y=w129) -> (x+y=w128:dbl)
        n155 = Square Root(x=w128) -> (sqrt(x)=w127:dbl)
        "delta_distance" <- w127
        n156 = Divide(x=w105, y=w104) -> (x/y=w103:dbl)
        "tan(v)" <- w103
        n157 = Divide(x=w127, y=w109) -> (x/y=w108:dbl)
        "delta_velocity" <- w108
        n158 = Build Array (concatenate)(w102, w103) -> (w101:dbl[])
        n159 = Build Array (concatenate) "delta_velocity"(w107, w108) -> (w106:dbl[])
        n160 = Build Array(w159, w158, w157, w156, w151, w155, w154, w153, w147, w143, w124, w123, w110, w106, w101, w93) -> (→"all parameters":dbl[][])
        "Numeric 5" <- w81
        "T" <- w81
        "T" <- w81
        "prev_end_point_x" <- w139
        "prev_end_point_y" <- w135
        "prev time" <- w118
      }
    }
    frame #3 {
      # "4. The error -314220 indicates that the other endpoint has been destroyed. The VI ignores this error."
      # "3. Destroy the stream endpoint when you click Stop or when an error occurs."
      # "Close"
      n161 = Flush Stream(8:w376, 11:w379) -> (0:w377:errorcluster, 3:w378:refnum<k21>)  [unwired: 2 in, 1 out]
      n162 = Destroy Stream Endpoint(8:w377, 11:w378) -> (0:w371:errorcluster)
      n163 = Unbundle By Name(w371) -> ("code"=w375:i32)
      n164 = xnode "Error Ring"() -> ("错误输出"=w372:errorcluster)
      n165 = Not Equal?(x=w375, y=-314220) -> (x != y?=w373:bool)
      n166 = Select(t=w371, s=w373, f=w372) -> (s? t:f=→"error out":errorcluster)
    }
  }
